vi "PPSU 2 Queue.vi"(7 "Option":T1(ring)=enum."Close", 8 "error in":errorcluster, 10 "Messages":cluster{"Message":string, "Data":variant}[](array[cluster]), 11 "Message":cluster{"Message":string, "Data":variant}) -> (0 "error out":errorcluster, 3 "Message Out":cluster{"Message":string, "Data":variant})   [LabVIEW 2022 SP3]
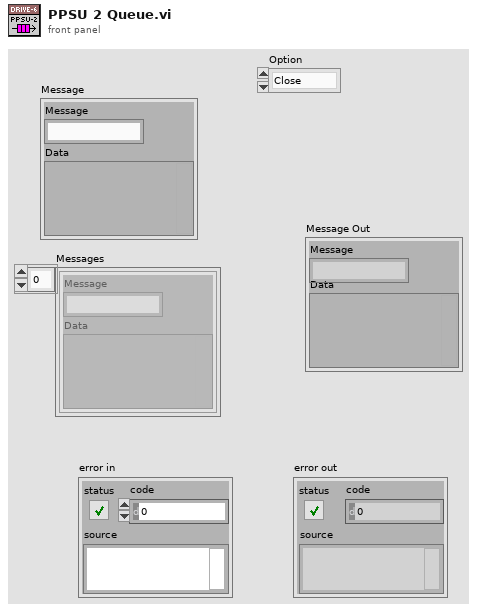
[diagram p1: front panel]
types:
  T1 = enum16{"Init", "EnQ '1'", "EnQ 'n'", "EnQ Opp", "DeQ", "Flush", "Close"}
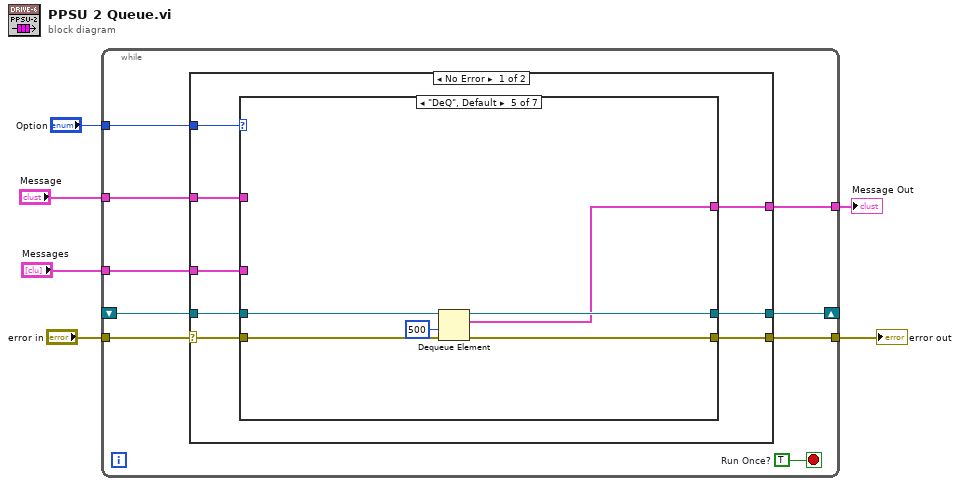
[diagram p0: block diagram]
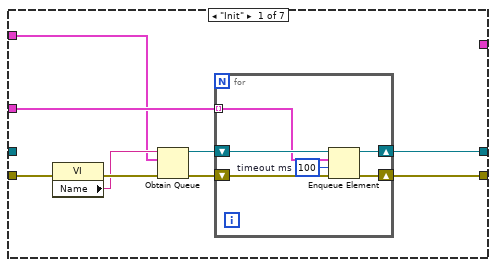
[diagram p2: hidden frame]
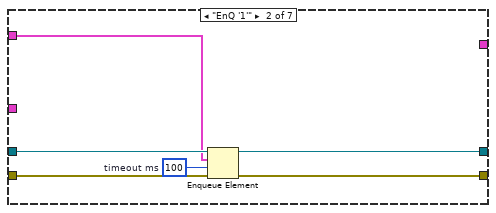
[diagram p3: hidden frame]
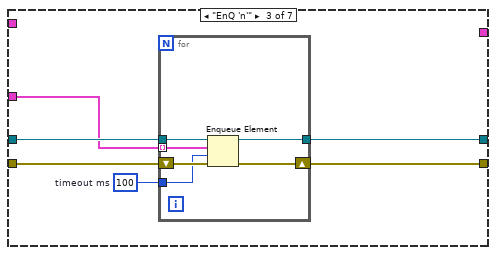
[diagram p4: hidden frame]
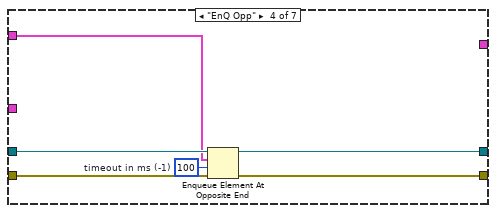
[diagram p5: hidden frame]
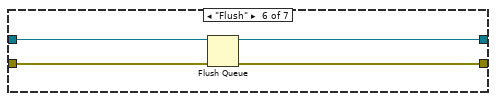
[diagram p6: hidden frame]
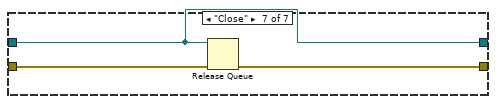
[diagram p7: hidden frame]
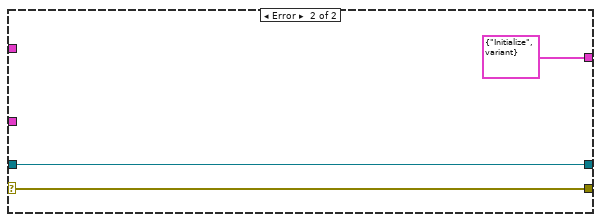
[diagram p8: hidden frame]
diagram:
  n1 = while {
    tunnel: "Option" -> [w15]
    tunnel: "error in" -> [w14]
    tunnel: "Message" -> [w13]
    tunnel: "Messages" -> [w12]
    tunnel: [w10] -> w4
    shift-right: [w9] -> _
    shift-left: _ -> [w8]
    tunnel: [w7] -> w1
    stop <- w11 stop-if-true
    w11 = TRUE  # Run Once?
    n2 = case shown="No Error" w14 {
      selector: w14 -> [w22 w77]
      tunnel: w15 -> [w23 _]
      tunnel: w13 -> [w21 _]
      tunnel: w12 -> [w20 _]
      tunnel: [w19 w77] -> w10
      tunnel: [w18 w78] -> w9
      tunnel: w8 -> [w17 w78]
      tunnel: [w16 cluster{"Message":string, "Data":variant} {"Message"="Initialize", "Data"=variant} ("Message")] -> w7
      frame No Error {
        n3 = case shown="\"DeQ\", Default" w23 {
          tunnel: w22 -> [w27 w44 w50 w62 w68 w69 w74]
          tunnel: w21 -> [w24 w41 _ w57 _ _ _]
          tunnel: w20 -> [w30 _ w46 _ _ _ _]
          tunnel: [w29 w43 w49 w61 w67 w72 w75] -> w19
          tunnel: [w28 w40 w47 w59 w65 w70 w73] -> w18
          tunnel: w17 -> [_ w42 w48 w60 w66 w71 w73]
          tunnel: [_ _ _ _ w64 _ _] -> w16
          frame "Init" {
            n4 = property class="VI"(error in=w27) -> (error out=w26:errorcluster, "Name"=w25:string)  [unwired: 1 in, 1 out]
            n5 = Obtain Queue(name (unnamed)=w25, element data type=w24, error in (no error)=w26) -> (queue out=w31:refnum<queue>, error out=w32:errorcluster)  [unwired: 2 in, 1 out]
            n6 = for {
              tunnel: w30 -> [w36] mode=indexing
              shift-right: [w35] -> w29
              shift-left: w32 -> [w38]
              shift-right: [w34] -> w28
              shift-left: w31 -> [w37]
              w33 = 100  # timeout ms
              n7 = Enqueue Element(queue=w37, element=w36, timeout in ms (-1)=w33, error in (no error)=w38) -> (queue out=w34:refnum<queue>, error out=w35:errorcluster)  [unwired: 1 out]
            }
          }
          frame "EnQ '1'" {
            w39 = 100  # timeout ms
            n8 = Enqueue Element(queue=w42, element=w41, timeout in ms (-1)=w39, error in (no error)=w44) -> (queue out=w40:refnum<queue>, error out=w43:errorcluster)  [unwired: 1 out]
          }
          frame "EnQ 'n'" {
            w45 = 100  # timeout ms
            n9 = for {
              tunnel: w48 -> [w54]
              tunnel: w46 -> [w53] mode=indexing
              tunnel: [w52] -> w47
              shift-right: [w55] -> w49
              shift-left: w50 -> [w56]
              tunnel: w45 -> [w51]
              n10 = Enqueue Element(queue=w54, element=w53, timeout in ms (-1)=w51, error in (no error)=w56) -> (queue out=w52:refnum<queue>, error out=w55:errorcluster)  [unwired: 1 out]
            }
          }
          frame "EnQ Opp" {
            w58 = 100  # timeout in ms (-1)
            n11 = Enqueue Element At Opposite End(queue=w60, element=w57, timeout in ms (-1)=w58, error in (no error)=w62) -> (queue out=w59:refnum<queue>, error out=w61:errorcluster)  [unwired: 1 out]
          }
          frame "DeQ", Default {
            n12 = Dequeue Element(queue=w66, timeout in ms (-1)=500, error in (no error)=w68) -> (queue out=w65:refnum<queue>, element=w64:cluster{"Message":string, "Data":variant}, error out=w67:errorcluster)  [unwired: 1 out]
          }
          frame "Flush" {
            n13 = Flush Queue(queue=w71, error in (no error)=w69) -> (queue out=w70:refnum<queue>, error out=w72:errorcluster)  [unwired: 1 out]
          }
          frame "Close" {
            n14 = Release Queue(queue=w73, error in (no error)=w74) -> (error out=w75:errorcluster)  [unwired: 1 in, 2 out]
          }
        }
      }
      frame Error {
      }
    }
  }
  "error out" <- w4
  "Message Out" <- w1
